vi "Send_Front_Panel_Config_to_Loops.vi"(5 "ClusterIn":T1={"Admin"={"Lvl"=enum."Admin", "Pwd"=""}, "RTConfig"={"Arm"=FALSE, "Number"=0.0, "String"=""}, "SMS"={"Enbl?"=FALSE, "Addr"=[]}, "FPGA"={"Target"=enum."4", "Channel"=enum."1", "Ref1"=refnum, "Ref2"=refnum}, "Config"={"UsrCfg"={"Paths"={"CfgFile"=path "", "LogFolder"=path "", "LogFile"=path "", "NAS path"=path "", "ThreshFile"=path "", "RedunFolder"=path ""}, "SampleRate"=0.0}, "FP_User"={"#NoiseSums"=0, "Max_df"=1, "AvgAvg"=FALSE, "#Avg"=0, "AutoCenter"=FALSE, "Inclin"={"Vmin"=0.0, "Vmax"=0.0, "Angle_min"=0.0, "Angle_max"=0.0, "Offset"=0.0, "Pos_Neg"=FALSE}, "1"={"Cal_"={"Fine"=0.0, "Coarse_"=0.0}, "Beac"={"Fine"=0.0, "Coarse_"=0.0}, "Scale"={"Step4"=0.0, "Step5"=0.0, "Step6"=0.0, "Step7"=0.0}, "Offset"=0.0, "Scale_Noise"=0.0, "Scale_Step1"=0.0, "Scale_In_RT"=0.0, "ScaleMeas"=0.0, "FreqsToRemove"=[], "Width"=[0, 1633], "ScaleMeasEnum"=enum."1", "FilterEnab"=enum."Step 1"}, "2"={"Cal_"={"Fine"=0.0, "Coarse_"=0.0}, "Beac"={"Fine"=0.0, "Coarse_"=0.0}, "Scale"={"Step4"=0.0, "Step5"=0.0, "Step6"=0.0, "Step7"=0.0}, "Offset"=0.0, "Scale_Noise"=0.0, "Scale_Step1"=0.0, "Scale_In_RT"=0.0, "ScaleMeas"=0.0, "FreqsToRemove"=[], "Width"=[0, 1633], "ScaleMeasEnum"=enum."1", "FilterEnab"=enum."Step 1"}, "3"={"Cal_"={"Fine"=0.0, "Coarse_"=0.0}, "Beac"={"Fine"=0.0, "Coarse_"=0.0}, "Scale"={"Step4"=0.0, "Step5"=0.0, "Step6"=0.0, "Step7"=0.0}, "Offset"=0.0, "Scale_Noise"=0.0, "Scale_Step1"=0.0, "Scale_In_RT"=0.0, "ScaleMeas"=0.0, "FreqsToRemove"=[], "Width"=[0, 1633], "ScaleMeasEnum"=enum."1", "FilterEnab"=enum."Step 1"}, "4"={"Cal_"={"Fine"=0.0, "Coarse_"=0.0}, "Beac"={"Fine"=0.0, "Coarse_"=0.0}, "Scale"={"Step4"=0.0, "Step5"=0.0, "Step6"=0.0, "Step7"=0.0}, "Offset"=0.0, "Scale_Noise"=0.0, "Scale_Step1"=0.0, "Scale_In_RT"=0.0, "ScaleMeas"=0.0, "FreqsToRemove"=[], "Width"=[0, 1633], "ScaleMeasEnum"=enum."1", "FilterEnab"=enum."Step 1"}, "Target to Probe"=enum."4", "SNR_Thresh"=1.0, "Paths"={"CfgFile"=path "", "LogFolder"=path "", "LogFile"=path "", "NAS path"=path "", "ThreshFile"=path "", "RedunFolder"=path ""}, "Connex_Location"="", "SimulateFPGA"=FALSE, "Deadband"=0.0}}, "Stat"={"SysState"=enum."Init", "TrackRate"=FALSE, "AutoCentr"=FALSE}, "Alarm"={"TC13"={"Enbl"=FALSE, "ErrsAndWarns"={0.0, 5.663716814159292, 7.168141592920354, 8.584070796460177}}, "AI1"={"Enbl"=FALSE, "ErrsAndWarns"={0.0, 5.663716814159292, 7.168141592920354, 8.584070796460177}}, "AI2"={"Enbl"=FALSE, "ErrsAndWarns"={0.0, 5.663716814159292, 7.168141592920354, 8.584070796460177}}, "AI3"={"Enbl"=FALSE, "ErrsAndWarns"={0.0, 5.663716814159292, 7.168141592920354, 8.584070796460177}}, "AI4"={"Enbl"=FALSE, "ErrsAndWarns"={0.0, 5.663716814159292, 7.168141592920354, 8.584070796460177}}, "AI5"={"Enbl"=FALSE, "ErrsAndWarns"={0.0, 5.663716814159292, 7.168141592920354, 8.584070796460177}}, "AI6"={"Enbl"=FALSE, "ErrsAndWarns"={0.0, 5.663716814159292, 7.168141592920354, 8.584070796460177}}, "AI18"={"Enbl"=FALSE, "ErrsAndWarns"={0.0, 5.663716814159292, 7.168141592920354, 8.584070796460177}}, "AI19"={"Enbl"=FALSE, "ErrsAndWarns"={0.0, 5.663716814159292, 7.168141592920354, 8.584070796460177}}, "TE1"={"Enbl"=FALSE, "ErrsAndWarns"={0.0, 5.663716814159292, 7.168141592920354, 8.584070796460177}}, "TE2"={"Enbl"=TRUE, "ErrsAndWarns"={0.0, 5.663716814159292, 7.168141592920354, 8.584070796460177}}, "TE3"={"Enbl"=FALSE, "ErrsAndWarns"={0.0, 5.663716814159292, 7.168141592920354, 8.584070796460177}}, "ADAM1"={"Enbl"=FALSE, "ErrsAndWarns"={0.0, 5.663716814159292, 7.168141592920354, 8.584070796460177}}, "ADAM2"={"Enbl"=FALSE, "ErrsAndWarns"={0.0, 5.663716814159292, 7.168141592920354, 8.584070796460177}}, "ADAM3"={"Enbl"=FALSE, "ErrsAndWarns"={0.0, 5.663716814159292, 7.168141592920354, 8.584070796460177}}, "ADAM4"={"Enbl"=FALSE, "ErrsAndWarns"={0.0, 5.663716814159292, 7.168141592920354, 8.584070796460177}}, "72CoBeacFreq"={"Enbl"=FALSE, "ErrsAndWarns"={0.0, 5.663716814159292, 7.168141592920354, 8.584070796460177}}, "72CoCalFreq"={"Enbl"=FALSE, "ErrsAndWarns"={0.0, 5.663716814159292, 7.168141592920354, 8.584070796460177}}, "84CoBeacFreq"={"Enbl"=FALSE, "ErrsAndWarns"={0.0, 5.663716814159292, 7.168141592920354, 8.584070796460177}}, "84CoCalFreq"={"Enbl"=FALSE, "ErrsAndWarns"={0.0, 5.663716814159292, 7.168141592920354, 8.584070796460177}}, "72Co_CalTonePwr"={"Enbl"=FALSE, "ErrsAndWarns"={0.0, 5.663716814159292, 7.168141592920354, 8.584070796460177}}, "72X_CalTonePwr"={"Enbl"=FALSE, "ErrsAndWarns"={0.0, 5.663716814159292, 7.168141592920354, 8.584070796460177}}, "84Co_CalTonePwr"={"Enbl"=FALSE, "ErrsAndWarns"={0.0, 5.663716814159292, 7.168141592920354, 8.584070796460177}}, "84X_CalTonePwr"={"Enbl"=FALSE, "ErrsAndWarns"={0.0, 5.663716814159292, 7.168141592920354, 8.584070796460177}}}} {"Alarm"."84X_CalTonePwr"."ErrsAndWarns" scale=-120.0..-45.0; "Alarm"."72X_CalTonePwr"."ErrsAndWarns" scale=-120.0..-45.0; "Alarm"."84Co_CalTonePwr"."ErrsAndWarns" scale=-120.0..-45.0; "Alarm"."72Co_CalTonePwr"."ErrsAndWarns" scale=-120.0..-45.0; "Alarm"."84CoCalFreq"."ErrsAndWarns" scale=24.9..25.1; "Alarm"."84CoBeacFreq"."ErrsAndWarns" scale=25.5..27.0; "Alarm"."72CoCalFreq"."ErrsAndWarns" scale=24.9..25.1; "Alarm"."72CoBeacFreq"."ErrsAndWarns" scale=25.5..27.0; "Alarm"."ADAM4"."ErrsAndWarns" scale=30.0..52.0; "Alarm"."ADAM3"."ErrsAndWarns" scale=30.0..52.0; "Alarm"."ADAM2"."ErrsAndWarns" scale=30.0..52.0; "Alarm"."ADAM1"."ErrsAndWarns" scale=30.0..52.0; "Alarm"."TE3"."ErrsAndWarns" scale=30.0..52.0; "Alarm"."TE2"."ErrsAndWarns" scale=30.0..52.0; "Alarm"."TE1"."ErrsAndWarns" scale=20.0..52.0; "Alarm"."AI19"."ErrsAndWarns" scale=0.0..60.0; "Alarm"."AI18"."ErrsAndWarns" scale=-10.0..10.0; "Alarm"."AI6"."ErrsAndWarns" scale=0.0..35.0; "Alarm"."AI5"."ErrsAndWarns" scale=0.0..20.0; "Alarm"."AI4"."ErrsAndWarns" scale=0.0..15.0; "Alarm"."AI3"."ErrsAndWarns" scale=0.0..10.0; "Alarm"."AI2"."ErrsAndWarns" scale=0.0..10.0; "Alarm"."TC13"."ErrsAndWarns" scale=-10.0..40.0; "Config"."FP_User"."Deadband" format="%#.0f"}, 6 "Log_Q":refnum<queue>, 8 "error in (no error)":errorcluster, 9 "Noise_Q":refnum<queue>, 10 "Tones_Q":refnum<queue>) -> (0 "error out":errorcluster)   [LabVIEW 2018]
doc: "Send user config to HW loop, Tones Loop, Noise Floor Loop, and Log Loop"
uses:
  Controls/Enums/NoiseQueueElements.ctl
  Queue/DataQueueElements.ctl
  Controls/MasterCluster.ctl
  Controls/Clusts/AdminCluster.ctl
  Controls/UserLevelEnum.ctl
  Controls/RT_Config.ctl
  Controls/SMSDataCluster.ctl
  Controls/Clusts/FPGA_Config_Clust.ctl
  Controls/Enums/TargetNumber.ctl
  Controls/Clusts/Config_Clust.ctl
  Controls/Clusts/UserConfig.ctl
  Controls/PathsCluster.ctl
  Controls/Clusts/FrontPanel_UserConfig.ctl
  Controls/Clusts/Inclinometer_User_Cfg.ctl
  Controls/Clusts/FP_UserTargetConfig.ctl
  Controls/Clusts/FreqShift.ctl
  Controls/Clusts/FPGA_Scale.ctl
  Controls/Enums/ScaleMeasure.ctl
  Controls/RadioButtons/FilterEnableRadio.ctl
  Controls/SystemStatusCluster.ctl
  Controls/SystemStateEnum.ctl
  Controls/Clusts/AlarmSettingsClust.ctl
  Controls/Clusts/AlarmThresh_OneChan.ctl
  Controls/Enums/LogLoopEnum.ctl
  Controls/Enums/AI_Loop_Enum.ctl
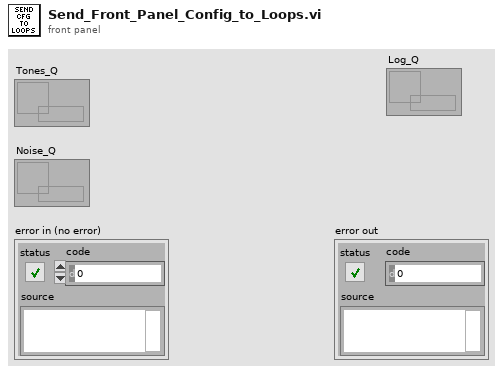
[diagram p1: front panel]
types:
  T1 = typedef "MasterCluster.ctl" = cluster{"Admin":T2, "RTConfig":T4, "SMS":T5, "FPGA":T6, "Config":T8, "Stat":T18, "Alarm":T20}
  T2 = typedef "AdminCluster.ctl" = cluster{"Lvl":T3, "Pwd":string}
  T3 = typedef "UserLevelEnum.ctl" = enum16{"Admin", "Operator"}
  T4 = typedef "RT_Config.ctl" = cluster{"Arm":bool, "Number":dbl, "String":string}
  T5 = typedef "SMSDataCluster.ctl" = cluster{"Enbl?":bool, "Addr":string[]}
  T6 = typedef "FPGA_Config_Clust.ctl" = cluster{"Target":T7, "Channel":T7, "Ref1":refnum<k20>, "Ref2":refnum<k20>}
  T7 = typedef "TargetNumber.ctl" = enum16{"1", "2", "3", "4"}
  T8 = typedef "Config_Clust.ctl" = cluster{"UsrCfg":T9, "FP_User":T11}
  T9 = typedef "UserConfig.ctl" = cluster{"Paths":T10, "SampleRate":dbl}
  T10 = typedef "PathsCluster.ctl" = cluster{"CfgFile":path, "LogFolder":path, "LogFile":path, "NAS path":path, "ThreshFile":path, "RedunFolder":path}
  T11 = typedef "FrontPanel_UserConfig.ctl" = cluster{"#NoiseSums":u32, "Max_df":u32, "AvgAvg":bool, "#Avg":u16, "AutoCenter":bool, "Inclin":T12, "1":T13, "2":T13, "3":T13, "4":T13, "Target to Probe":T7, "SNR_Thresh":dbl, "Paths":T10, "Connex_Location":string, "SimulateFPGA":bool, "Deadband":dbl}
  T12 = typedef "Inclinometer_User_Cfg.ctl" = cluster{"Vmin":dbl, "Vmax":dbl, "Angle_min":dbl, "Angle_max":dbl, "Offset":dbl, "Pos_Neg":bool}
  T13 = typedef "FP_UserTargetConfig.ctl" = cluster{"Cal_":T14, "Beac":T14, "Scale":T15, "Offset":fxp<+/-,16,16>, "Scale_Noise":fxp<+/-,30,30>, "Scale_Step1":fxp<+/-,17,17>, "Scale_In_RT":ext, "ScaleMeas":fxp<+/-,16,1>, "FreqsToRemove":i32[], "Width":i32[], "ScaleMeasEnum":T16, "FilterEnab":T17}
  T14 = typedef "FreqShift.ctl" = cluster{"Fine":dbl, "Coarse_":dbl}
  T15 = typedef "FPGA_Scale.ctl" = cluster{"Step4":fxp<+/-,23,23>, "Step5":fxp<+/-,23,23>, "Step6":fxp<+/-,23,23>, "Step7":fxp<+/-,23,23>}
  T16 = typedef "ScaleMeasure.ctl" = enum16{"1", "10", "50", "42"}
  T17 = typedef "FilterEnableRadio.ctl" = enum32{"None", "Step 1", "Frequency Shift", "Step 4", "Step 5", "Step 6", "Step 7"}
  T18 = typedef "SystemStatusCluster.ctl" = cluster{"SysState":T19, "TrackRate":bool, "AutoCentr":bool}
  T19 = typedef "SystemStateEnum.ctl" = enum16{"Init", "Idle", "Running", "System Fault", "System Error", "Exit"}
  T20 = typedef "AlarmSettingsClust.ctl" = cluster{"TC13":T21, "AI1":T21, "AI2":T21, "AI3":T21, "AI4":T21, "AI5":T21, "AI6":T21, "AI18":T21, "AI19":T21, "TE1":T21, "TE2":T21, "TE3":T21, "ADAM1":T21, "ADAM2":T21, "ADAM3":T21, "ADAM4":T21, "72CoBeacFreq":T21, "72CoCalFreq":T21, "84CoBeacFreq":T21, "84CoCalFreq":T21, "72Co_CalTonePwr":T21, "72X_CalTonePwr":T21, "84Co_CalTonePwr":T21, "84X_CalTonePwr":T21}
  T21 = typedef "AlarmThresh_OneChan.ctl" = cluster{"Enbl":bool, "ErrsAndWarns":cluster{dbl, dbl, dbl, dbl}}
  T22 = typedef "AI_Loop_Enum.ctl" = enum16{"AI_Init", "AI_Config", "AI_Alarm", "AI_Read", "AI_ChkTime", "AI_Exit"}
  T23 = typedef "LogLoopEnum.ctl" = enum16{"Log_Init", "Log_Config", "Log_CfgAlarm", "Log_TimeDomain", "Log_Tone", "Log_NoiseTrace", "Log_NoiseSum", "Log_DO", "Log_AI", "Log_TC", "Log_Disdrom", "Log_Weather", "Log_TE", "Log_ADAM", "Log_UPS", "Log_ChkTime", "Log_Alarm", "Log_SSH", "Log_Write", "Log_Exit"}
  T24 = typedef "NoiseQueueElements.ctl" = enum16{"Noise_Startup", "Noise_Init", "Noise_Macro", "Noise_Config", "Noise_NewData", "Noise_Transform", "Noise_SumdTrace", "Noise_Send", "Noise_Probes", "Noise_Exit"}
  T25 = typedef "DataQueueElements.ctl" = enum16{"Data_Init", "Data_Config", "Data_AddData", "Data_FreqShift", "Data_FPGA_Write", "Data_Transform", "Data_Send", "Data_Exit"}
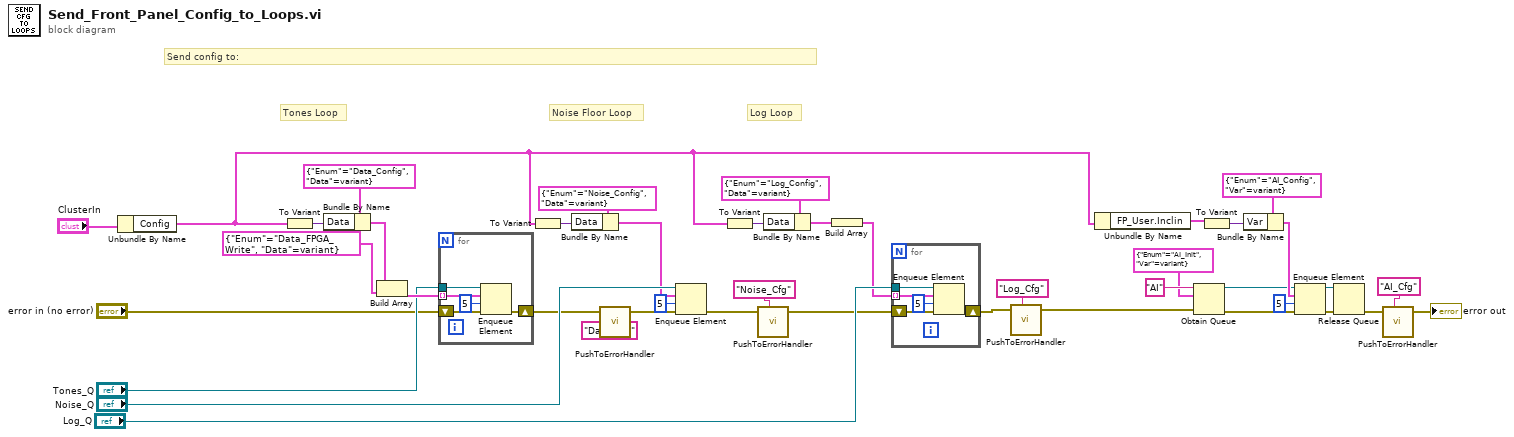
[diagram p0: block diagram]
diagram:
  # "Log Loop"
  # "Noise Floor Loop"
  # "Tones Loop"
  # "Send config to:"
  n1 = Unbundle By Name("ClusterIn") -> ("Config"=w2:T8)
  n2 = To Variant(anything=w2) -> (Variant=w33:variant)
  n3 = Bundle By Name(cluster=cluster{"Enum":T25, "Data":variant} {"Enum"=enum."Data_Config", "Data"=variant} ("element"), "Data"=w33) -> (w36:cluster{"Enum":T25, "Data":variant})
  n4 = Build Array(w36, cluster{"Enum":T25, "Data":variant} {"Enum"=enum."Data_FPGA_Write", "Data"=variant} ("element")) -> (w37:cluster{"Enum":T25, "Data":variant}[])
  n5 = for {
    tunnel: "Tones_Q" -> [w45]
    tunnel: w37 -> [w44] mode=indexing
    shift-right: [w46] -> w12
    shift-left: "error in (no error)" -> [w47]
    n6 = Enqueue Element(queue=w45, element=w44, timeout in ms (-1)=5, error in (no error)=w47) -> (error out=w46:errorcluster)  [unwired: 2 out]
  }
  n7 = To Variant(anything=w2) -> (Variant=w42:variant)
  n8 = Bundle By Name(cluster=cluster{"Enum":T24, "Data":variant} {"Enum"=enum."Noise_Config", "Data"=variant}, "Data"=w42) -> (w40:cluster{"Enum":T24, "Data":variant})
  n9 = call "PushToErrorHandler.vi"("ErrorIn"=w12, "ErrorLocation"="Data_Cfg") -> ("ErrorOut"=w11:errorcluster)  [unwired: 5 in]
  n10 = Enqueue Element(queue="Noise_Q", element=w40, timeout in ms (-1)=5, error in (no error)=w11) -> (error out=w10:errorcluster)  [unwired: 2 out]
  n11 = To Variant(anything=w2) -> (Variant=w30:variant)
  n12 = call "PushToErrorHandler.vi"("ErrorIn"=w10, "ErrorLocation"="Noise_Cfg") -> ("ErrorOut"=w9:errorcluster)  [unwired: 5 in]
  n13 = Bundle By Name(cluster=cluster{"Enum":T23, "Data":variant} {"Enum"=enum."Log_Config", "Data"=variant} ("element"), "Data"=w30) -> (w28:cluster{"Enum":T23, "Data":variant})
  n14 = Build Array(w28) -> (w27:cluster{"Enum":T23, "Data":variant}[])
  n15 = for {
    tunnel: "Log_Q" -> [w50]
    shift-right: [w51] -> w8
    shift-left: w9 -> [w52]
    tunnel: w27 -> [w49] mode=indexing
    n16 = Enqueue Element(queue=w50, element=w49, timeout in ms (-1)=5, error in (no error)=w52) -> (error out=w51:errorcluster)  [unwired: 2 out]
  }
  n17 = call "PushToErrorHandler.vi"("ErrorIn"=w8, "ErrorLocation"="Log_Cfg") -> ("ErrorOut"=w3:errorcluster)  [unwired: 5 in]
  n18 = Unbundle By Name(w2) -> ("FP_User.Inclin"=w24:T12)
  n19 = Obtain Queue(name (unnamed)="AI", element data type=cluster{"Enum":T22, "Var":variant} {"Enum"=enum."AI_Init", "Var"=variant}, error in (no error)=w3) -> (queue out=w20:refnum<queue>, error out=w21:errorcluster)  [unwired: 2 in, 1 out]
  n20 = To Variant(anything=w24) -> (Variant=w26:variant)
  n21 = Bundle By Name(cluster=cluster{"Enum":T22, "Var":variant} {"Enum"=enum."AI_Config", "Var"=variant}, "Var"=w26) -> (w23:cluster{"Enum":T22, "Var":variant})
  n22 = Enqueue Element(queue=w20, element=w23, timeout in ms (-1)=5, error in (no error)=w21) -> (queue out=w19:refnum<queue>, error out=w22:errorcluster)  [unwired: 1 out]
  n23 = Release Queue(queue=w19, error in (no error)=w22) -> (error out=w7:errorcluster)  [unwired: 1 in, 2 out]
  n24 = call "PushToErrorHandler.vi"("ErrorIn"=w7, "ErrorLocation"="AI_Cfg") -> ("ErrorOut"=→"error out":errorcluster)  [unwired: 5 in]
